vi "DOCK_MAIN_get_current_size_and_part_number.vi"(8 "error_in":errorcluster, 11 "batch_ID":string) -> (0 "error_out":errorcluster, 2 "part_number":string, 3 "current_size":u16)   [LabVIEW 2019]
uses:
  FGV/SQL_connection/FGV_DOCK_SQL_connection.ctl
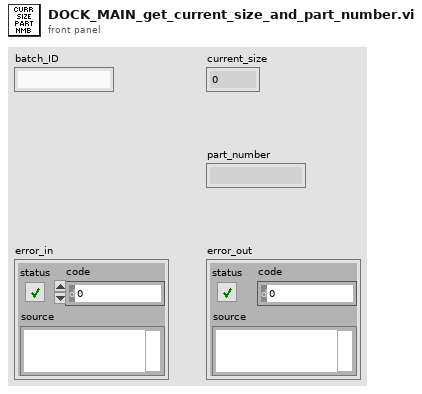
[diagram p1: front panel]
types:
  T1 = typedef "FGV_DOCK_SQL_connection.ctl" = enum16{"initialize", "connect", "read_tables", "read_columns", "SELECT", "INSERT", "UPDATE", "DELETE", "EXEC + headers", "EXEC", "TRANSACTION", "connection_active?", "disconnect"}
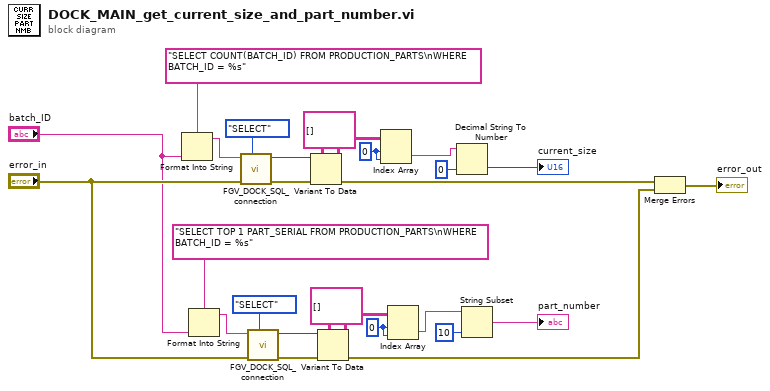
[diagram p0: block diagram]
diagram:
  w15 = 0 ("index (row)")
  w24 = 0 ("index (row)")
  n1 = Format Into String(format string="SELECT COUNT(BATCH_ID) FROM PRODUCTION_PARTS\nWHERE BATCH_ID = %s", "batch_ID") -> (resulting string=w26:string)  [unwired: 2 in, 1 out]
  n2 = Format Into String(format string="SELECT TOP 1 PART_SERIAL FROM PRODUCTION_PARTS\nWHERE BATCH_ID = %s", "batch_ID") -> (resulting string=w13:string)  [unwired: 2 in, 1 out]
  n3 = call "FGV_DOCK_SQL_connection.vi"("options"=FGV_DOCK_SQL_connection."SELECT", "error_in"="error_in", "SQL_statement"=w26) -> ("error_out"=w27:errorcluster, "SQL_result"=w21:variant)  [unwired: 4 in, 3 out]
  n4 = call "FGV_DOCK_SQL_connection.vi"("options"=FGV_DOCK_SQL_connection."SELECT", "error_in"="error_in", "SQL_statement"=w13) -> ("error_out"=w10:errorcluster, "SQL_result"=w18:variant)  [unwired: 4 in, 3 out]
  n5 = Variant To Data(error in=w27, type=string[][] [], Variant=w21) -> (data=w23:string[][], error out=w9:errorcluster)
  n6 = Variant To Data(error in=w10, type=string[][] [], Variant=w18) -> (data=w16:string[][], error out=w7:errorcluster)
  n7 = Index Array(array=w23, index (row)=w24, index (col)=w24) -> (element=w2:string)
  n8 = Index Array(array=w16, index (row)=w15, index (col)=w15) -> (element=w6:string)
  n9 = Decimal String To Number(string=w2, default (0L)=u16 0 ("default (0 I32)")) -> (number=→"current_size":u16)  [unwired: 1 in, 1 out]
  n10 = String Subset(string=w6, length (rest)=10 ("length (rest)")) -> (substring=→"part_number":string)  [unwired: 1 in]
  n11 = Merge Errors(w9, w7) -> (→"error_out":errorcluster)
